vi "Pure Function Wrapper.vi"() -> ()   [LabVIEW 2019]
uses:
  <vilib>/Utility/miscctls.llb/LVMapReplaceAction.ctl
panel:
  out "Output Array":i32[](array[numeric])
  in  "Iterations":i32
  in  "Offset":i32
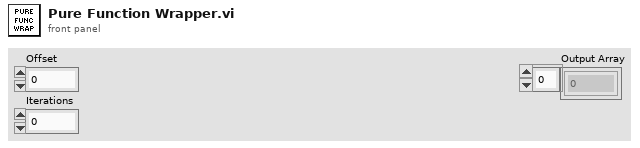
[diagram p1: front panel]
types:
  T1 = map{cluster{"Iterations":i32, "Offset":i32}, i32[]}
  T2 = typedef "LVMapReplaceAction.ctl" = enum32{"Modify Entry only if found", "Add or Modify Entry", "Delete Entry"}
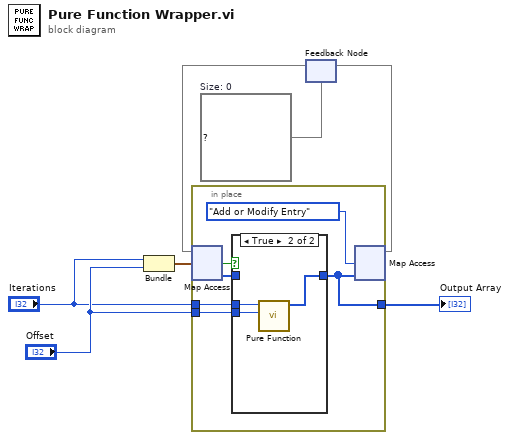
[diagram p0: block diagram]
diagram:
  w3 = T1 {}  # Size: 0
  n1 = Bundle("Iterations"="Iterations", "Offset"="Offset") -> (w4:cluster{"Iterations":i32, "Offset":i32})  [unwired: 1 in]
  n2 = feedback #1(w3) -> (w2:T1)
  n3 = in-place {
    in-place-border: "Offset" -> [w13]
    in-place-border: "Iterations" -> [w12]
    in-place-border: [w9] -> w7
    n4 = in-place-map #2(w2, w4) -> (w10:i32[], w11:bool)  [unwired: 1 in]
    n5 = case shown="True" w11 {
      tunnel: w13 -> [_ w17]
      tunnel: w12 -> [_ w16]
      tunnel: [w14 w15] -> w9
      tunnel: w10 -> [w14 _]
      frame False {
      }
      frame True {
        n6 = call "Pure Function.vi"("Offset"=w17, "Iterations"=w16) -> ("Output Array"=w15:i32[])  [unwired: 9 in]
      }
    }
    n7 = in-place-map #2(w9, LVMapReplaceAction."Add or Modify Entry" ("action")) -> (w1:T1)  [unwired: 2 out]
  }
  "Output Array" <- w7
  n8 = feedback-in #1(w1) -> ()
